vi "Single Class_Multiple_State_External [].vi"(0 "State#":i32=1000, 1 "State_Interval_Time(s)":dbl=0.001 min=0.0 max=86400.0 format="%#_13p", 2 "Time Target (s)":dbl=30.0 format="%#_13g", 3 "System_Delay(s)":dbl=0.01 min=0.0 max=86400.0 format="%#_13p") -> ()   [LabVIEW 2021]
uses:
  C:/Program Files (x86)/Hyper State Machine Framework/SSW_Hyper_State_Machine.lvlibp/State_Machine_Class/Main_State_Machine/Hyper_State_Machine.lvclass
  C:/Program Files (x86)/Hyper State Machine Framework/SSW_Hyper_State_Machine.lvlibp/State_Machine_Class/State_Machine_Module.llb/State Machine[].ctl
  C:/Program Files (x86)/Hyper State Machine Framework/SSW_Hyper_State_Machine.lvlibp/State_Machine_Class/State_Machine_Module.llb/Iterval.ctl
  C:/Program Files (x86)/Hyper State Machine Framework/SSW_Hyper_State_Machine.lvlibp/State_Machine_Class/State_Machine_Module.llb/Lock_Unlock.ctl
  C:/Program Files (x86)/Hyper State Machine Framework/SSW_Hyper_State_Machine.lvlibp
panel:
  in  "State[]":refnum<class "Hyper_State_Machine.lvclass">[](array[class])
  out "Current State":string
  out "Show_Stop_Button":bool=TRUE
  in  "Unlock":bool
  in  "Reset":bool
  in  "Lock Even":bool
  in  "Lock Odd":bool
  in  "lock All":bool
  in  "Stop":bool
  out "Timing":dbl[](array[numeric])
  out "Lock":bool[](array[boolean])
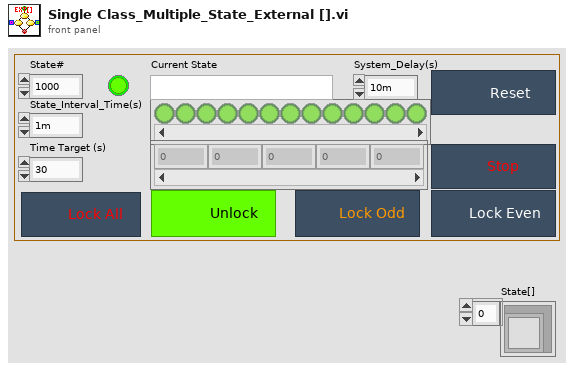
[diagram p1: front panel]
types:
  T1 = typedef "SSW_Hyper_State_Machine.lvlibp/State Machine.ctl" = cluster{"Command":string, "Data":variant}
  T2 = typedef "SSW_Hyper_State_Machine.lvlibp/State Machine[].ctl" = cluster{"Command":string, "Data":variant}[]
  T3 = typedef "SSW_Hyper_State_Machine.lvlibp/Lock_Unlock.ctl" = cluster{"Action_Mode (Get)":enum16{"Set", "Get"}, "Action_Set (False)":bool, "State_In (Wait)":string}
  T4 = typedef "SSW_Hyper_State_Machine.lvlibp/Iterval.ctl" = cluster{"Delay(s)":dbl, "State (Interval_Delay)":string}
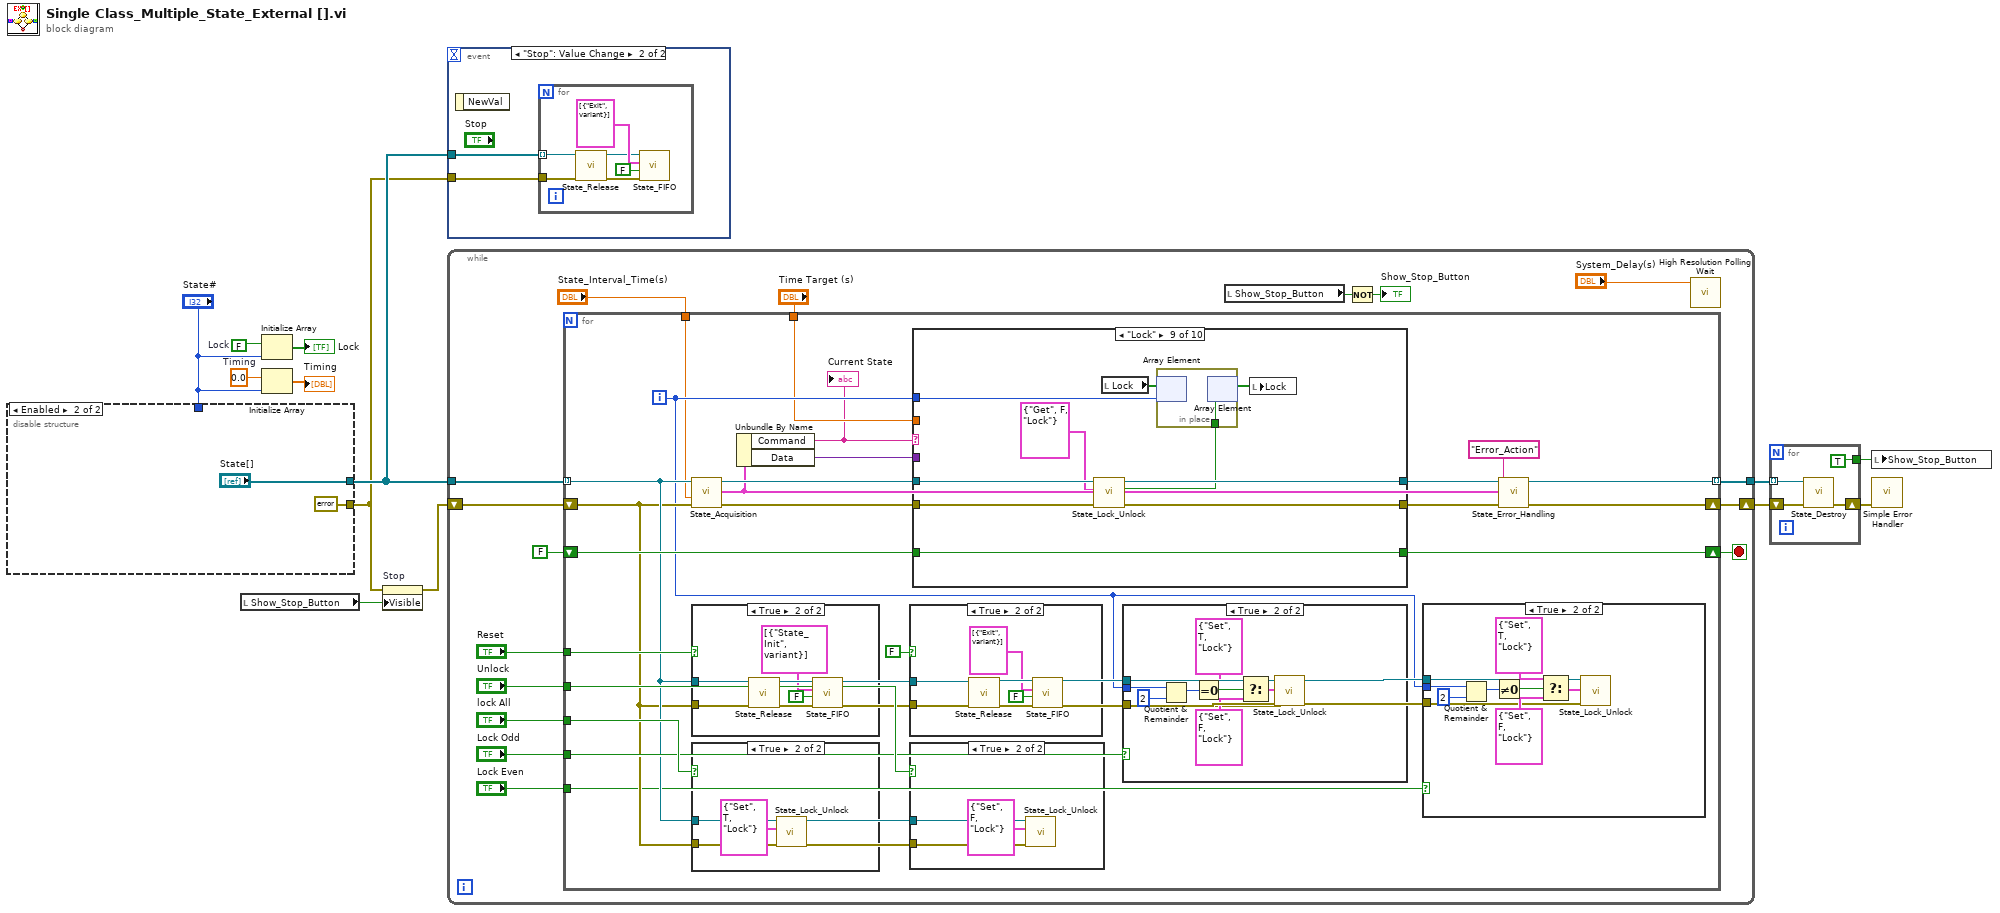
[diagram p0: block diagram]
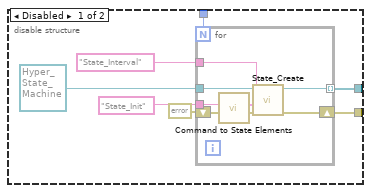
[diagram p2: hidden frame]
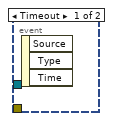
[diagram p3: hidden frame]
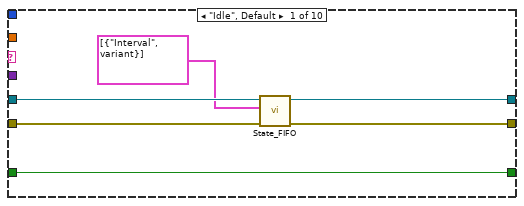
[diagram p10: hidden frame]
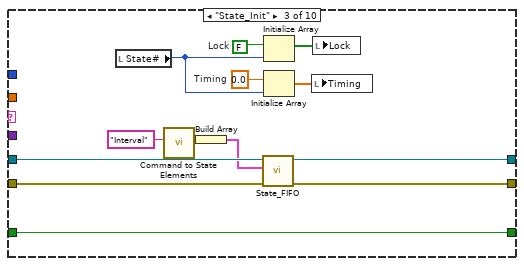
[diagram p12: hidden frame]
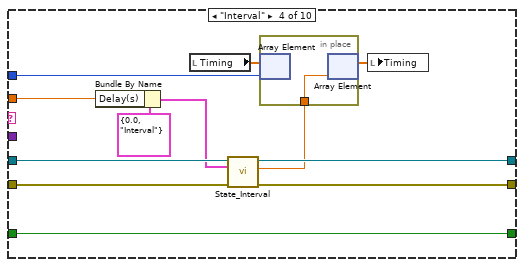
[diagram p13: hidden frame]
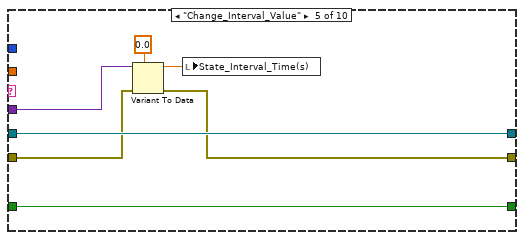
[diagram p14: hidden frame]
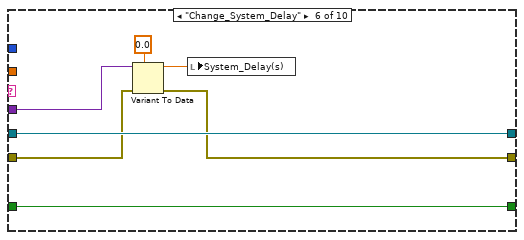
[diagram p15: hidden frame]
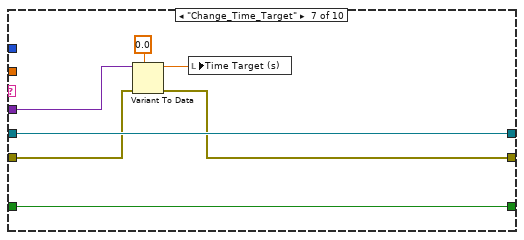
[diagram p16: hidden frame]
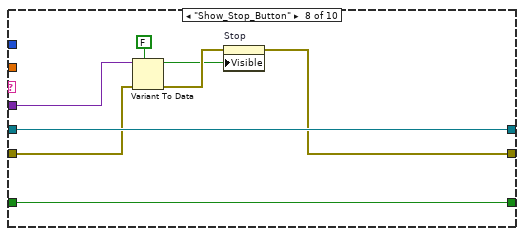
[diagram p17: hidden frame]
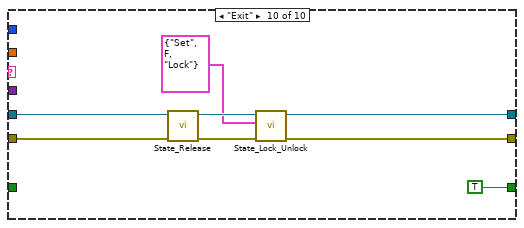
[diagram p18: hidden frame]
diagram:
  w10 = 0.0  # Timing
  w13 = FALSE  # Lock
  n1 = disable-structure shown="Enabled" {
    disable-tunnel: "State#" -> [w20 _]
    disable-tunnel: [w19 "State[]"] -> w2
    disable-tunnel: [w18 errorcluster {"status"=FALSE, "code"=0, "source"=""} ("error out")] -> w1
    frame Disabled {
      n2 = for {
        N: w20 -> [_]
        tunnel: refnum<class "Hyper_State_Machine.lvclass"> refnum ("SSW_Hyper_State_Machine.lvlibp:Hyper_State_Machine.lvclass") -> [w27]
        tunnel: "State_Init" ("Command") -> [w25]
        tunnel: "State_Interval" ("Core_Interval_Name(State_Interval)") -> [w24]
        shift-right: [w23] -> w18
        shift-left: errorcluster {"status"=FALSE, "code"=0, "source"=""} ("error out") -> [w22]
        tunnel: [w21] -> w19 mode=indexing
        n3 = call "Command to State Elements.vi"("Command"=w25) -> ("Command to State Elements"=w26:T1)  [unwired: 10 in]
        n4 = call-dynamic "State_Create.vi"("error in (no error)"=w22, "Init_State(Option)"=w26, "State_Interval_Name"=w24, "State_Machine_Class in"=w27) -> ("error out"=w23:errorcluster, "State_Machine_Class out"=w21:refnum<class "Hyper_State_Machine.lvclass">)  [unwired: 5 in, 1 out]
      }
    }
    frame Enabled {
    }
  }
  n5 = local read "Show_Stop_Button"() -> (w4:bool)
  n6 = Initialize Array(w13, "State#") -> (→"Lock":bool[])
  n7 = Initialize Array(w10, "State#") -> (→"Timing":dbl[])
  n8 = property on="Stop" class="Bool"(error in=w1, "Visible"=w4) -> (error out=w5:errorcluster)  [unwired: 1 in, 1 out]
  n9 = event shown="[1] \"Stop\": Value Change" {
    selector: _ -> [_ _]
    dyn-events: _ -> [_ _]
    timeout: _ -> [_ _]
    tunnel: w2 -> [_ w31]
    tunnel: w1 -> [_ w30]
    event Timeout {
      n10 = event-data() -> ()  [unwired: 1 in, 3 out]
    }
    event "Stop": Value Change {
      n11 = event-data() -> ()  [unwired: 1 in, 1 out]
      n12 = for {
        tunnel: w31 -> [w33] mode=indexing
        tunnel: w30 -> [w32]
        n13 = call-dynamic "State_Release.vi"("error in (no error)"=w32, "State_Machine_Class in"=w33) -> ("error out"=w35:errorcluster, "State_Machine_Class out"=w34:refnum<class "Hyper_State_Machine.lvclass">)  [unwired: 8 in]
        n14 = call-dynamic "State_FIFO.vi"("error in (no error)"=w35, "State_Interval(Enable)"=FALSE, "State Machine[]"=T2 [{"Command"="Exit", "Data"=variant}], "State_Machine_Class in"=w34) -> ()  [unwired: 6 in, 2 out]
      }
    }
  }
  n15 = while {
    tunnel: w2 -> [w53]
    tunnel: [w49] -> w7
    shift-right: [w48] -> w6
    shift-left: w5 -> [w52]
    stop <- w51 stop-if-true
    n16 = for {
      tunnel: w53 -> [w61] mode=indexing
      shift-right: [w73] -> w48
      shift-left: w52 -> [w60]
      shift-right: [w68] -> w51
      shift-left: FALSE -> [w67]
      tunnel: [w66] -> w49 mode=indexing
      tunnel: "Reset" -> [w65]
      tunnel: "lock All" -> [w64]
      tunnel: "Unlock" -> [w63]
      tunnel: "Lock Odd" -> [w62]
      tunnel: "Lock Even" -> [w59]
      tunnel: "Time Target (s)" -> [w57]
      tunnel: "State_Interval_Time(s)" -> [w56]
      i -> [w58]
      n17 = call-dynamic "State_Acquisition.vi"("error in (no error)"=w60, "State_Interval_Time(s)"=w56, "Main_Machine_State_Class in"=w61) -> ("error out"=w74:errorcluster, "State"=w72:T1, "Main_Machine_State_Class out"=w75:refnum<class "Hyper_State_Machine.lvclass">)  [unwired: 2 in, 4 out]
      n18 = case shown="True" w65 {
        tunnel: w61 -> [_ w112]
        tunnel: w60 -> [_ w108]
        frame False {
        }
        frame True {
          n19 = call-dynamic "State_Release.vi"("error in (no error)"=w108, "State_Machine_Class in"=w112) -> ("error out"=w110:errorcluster, "State_Machine_Class out"=w111:refnum<class "Hyper_State_Machine.lvclass">)  [unwired: 8 in]
          n20 = call-dynamic "State_FIFO.vi"("error in (no error)"=w110, "State_Interval(Enable)"=FALSE, "State Machine[]"=T2 [{"Command"="State_Init", "Data"=variant}], "State_Machine_Class in"=w111) -> ()  [unwired: 6 in, 2 out]
        }
      }
      n21 = case shown="True" w64 {
        tunnel: w61 -> [_ w100]
        tunnel: w60 -> [_ w99]
        frame False {
        }
        frame True {
          n22 = call-dynamic "State_Lock_Unlock.vi"("error in (no error)"=w99, "Parameter"=T3 {"Action_Mode (Get)"=enum."Set", "Action_Set (False)"=TRUE, "State_In (Wait)"="Lock"}, "State_Machine_Class in"=w100) -> ()  [unwired: 6 in, 3 out]
        }
      }
      n23 = Unbundle By Name(w72) -> ("Command"=w54:string, "Data"=w76:variant)
      "Current State" <- w54
      n24 = case shown="True" FALSE {
        tunnel: w61 -> [_ w106]
        tunnel: w60 -> [_ w102]
        frame False {
        }
        frame True {
          n25 = call-dynamic "State_Release.vi"("error in (no error)"=w102, "State_Machine_Class in"=w106) -> ("error out"=w104:errorcluster, "State_Machine_Class out"=w105:refnum<class "Hyper_State_Machine.lvclass">)  [unwired: 8 in]
          n26 = call-dynamic "State_FIFO.vi"("error in (no error)"=w104, "State_Interval(Enable)"=FALSE, "State Machine[]"=T2 [{"Command"="Exit", "Data"=variant}], "State_Machine_Class in"=w105) -> ()  [unwired: 6 in, 2 out]
        }
      }
      n27 = case shown="True" w63 {
        tunnel: w61 -> [_ w96]
        tunnel: w60 -> [_ w97]
        frame False {
        }
        frame True {
          n28 = call-dynamic "State_Lock_Unlock.vi"("error in (no error)"=w97, "Parameter"=T3 {"Action_Mode (Get)"=enum."Set", "Action_Set (False)"=FALSE, "State_In (Wait)"="Lock"}, "State_Machine_Class in"=w96) -> ()  [unwired: 6 in, 3 out]
        }
      }
      n29 = case shown="\"Lock\"" w54 {
        tunnel: w76 -> [_ _ _ _ w153 w160 w167 w175 _ _]
        tunnel: w75 -> [w117 w121 w133 w140 w154 w161 w168 w176 w186 w194]
        tunnel: w74 -> [w116 w120 w131 w139 w152 w159 w166 w174 w185 w193]
        tunnel: [w115 w121 w132 w137 w154 w161 w168 w176 w184 w190] -> w70
        tunnel: [w114 w120 w130 w136 w151 w158 w165 w169 w183 w189] -> w69
        tunnel: w58 -> [_ _ _ w146 _ _ _ _ w178 _]
        tunnel: [w118 w119 w134 w143 w149 w156 w163 w173 w181 TRUE] -> w68
        tunnel: w67 -> [w118 w119 w134 w143 w149 w156 w163 w173 w181 _]
        tunnel: w57 -> [_ _ _ w142 _ _ _ _ _ _]
        frame "Idle", Default {
          n30 = call-dynamic "State_FIFO.vi"("error in (no error)"=w116, "State Machine[]"=T2 [{"Command"="Interval", "Data"=variant}], "State_Machine_Class in"=w117) -> ("error out"=w114:errorcluster, "State_Machine_Class out"=w115:refnum<class "Hyper_State_Machine.lvclass">)  [unwired: 7 in]
        }
        frame "State_Interval" {
          # "Execute Every Define of State Interval Time"
        }
        frame "State_Init" {
          w126 = 0.0  # Timing
          w125 = FALSE  # Lock
          n31 = local read "State#"() -> (w124:i32)
          n32 = call "Command to State Elements.vi"("Command"="Interval") -> ("Command to State Elements"=w128:T1)  [unwired: 10 in]
          n33 = Build Array(w128) -> (w127:T1[])
          n34 = call-dynamic "State_FIFO.vi"("error in (no error)"=w131, "State Machine[]"=w127, "State_Machine_Class in"=w133) -> ("error out"=w130:errorcluster, "State_Machine_Class out"=w132:refnum<class "Hyper_State_Machine.lvclass">)  [unwired: 7 in]
          n35 = Initialize Array(w125, w124) -> (w122:bool[])
          n36 = Initialize Array(w126, w124) -> (w123:dbl[])
          n37 = local write "Timing"(w123) -> ()
          n38 = local write "Lock"(w122) -> ()
        }
        frame "Interval" {
          n39 = Bundle By Name(cluster=T4 {"Delay(s)"=0.0, "State (Interval_Delay)"="Interval"} ("Parameter"), "Delay(s)"=w142) -> (w138:T4)
          n40 = local read "Timing"() -> (w145:dbl[])
          n41 = call-dynamic "State_Interval.vi"("error in (no error)"=w139, "Parameter"=w138, "State_Machine_Class in"=w140) -> ("error out"=w136:errorcluster, "Elapsed Time(s)"=w135:dbl, "State_Machine_Class out"=w137:refnum<class "Hyper_State_Machine.lvclass">)  [unwired: 6 in]
          n42 = in-place {
            in-place-border: w135 -> [w147]
            n43 = in-place-array #1(w145, w146) -> ()  [unwired: 1 out]
            n44 = in-place-array #1(w147) -> (w144:dbl[])  [unwired: 1 out]
          }
          n45 = local write "Timing"(w144) -> ()
        }
        frame "Change_Interval_Value" {
          n46 = Variant To Data(error in=w152, type=0.0 ("Time Target (s)"), Variant=w153) -> (data=w148:dbl, error out=w151:errorcluster)
          n47 = local write "State_Interval_Time(s)"(w148) -> ()
        }
        frame "Change_System_Delay" {
          n48 = Variant To Data(error in=w159, type=0.0 ("Time Target (s)"), Variant=w160) -> (data=w155:dbl, error out=w158:errorcluster)
          n49 = local write "System_Delay(s)"(w155) -> ()
        }
        frame "Change_Time_Target" {
          n50 = Variant To Data(error in=w166, type=0.0 ("Time Target (s)"), Variant=w167) -> (data=w162:dbl, error out=w165:errorcluster)
          n51 = local write "Time Target (s)"(w162) -> ()
        }
        frame "Show_Stop_Button" {
          n52 = Variant To Data(error in=w174, type=FALSE, Variant=w175) -> (data=w170:bool, error out=w171:errorcluster)
          n53 = property on="Stop" class="Bool"(error in=w171, "Visible"=w170) -> (error out=w169:errorcluster)  [unwired: 1 in, 1 out]
        }
        frame "Lock" {
          n54 = call-dynamic "State_Lock_Unlock.vi"("error in (no error)"=w185, "Parameter"=T3 {"Action_Mode (Get)"=enum."Get", "Action_Set (False)"=FALSE, "State_In (Wait)"="Lock"}, "State_Machine_Class in"=w186) -> ("error out"=w183:errorcluster, "Action_Get"=w177:bool, "State_Machine_Class out"=w184:refnum<class "Hyper_State_Machine.lvclass">)  [unwired: 6 in]
          n55 = local read "Lock"() -> (w179:bool[])
          n56 = in-place {
            in-place-border: w177 -> [w187]
            n57 = in-place-array #2(w179, w178) -> ()  [unwired: 1 out]
            n58 = in-place-array #2(w187) -> (w180:bool[])  [unwired: 1 out]
          }
          n59 = local write "Lock"(w180) -> ()
        }
        frame "Exit" {
          n60 = call-dynamic "State_Release.vi"("error in (no error)"=w193, "State_Machine_Class in"=w194) -> ("error out"=w191:errorcluster, "State_Machine_Class out"=w192:refnum<class "Hyper_State_Machine.lvclass">)  [unwired: 8 in]
          n61 = call-dynamic "State_Lock_Unlock.vi"("error in (no error)"=w191, "Parameter"=T3 {"Action_Mode (Get)"=enum."Set", "Action_Set (False)"=FALSE, "State_In (Wait)"="Lock"}, "State_Machine_Class in"=w192) -> ("error out"=w189:errorcluster, "State_Machine_Class out"=w190:refnum<class "Hyper_State_Machine.lvclass">)  [unwired: 6 in, 1 out]
        }
      }
      n62 = case shown="True" w62 {
        tunnel: w58 -> [_ w88]
        tunnel: w61 -> [_ w87]
        tunnel: w60 -> [_ w86]
        frame False {
        }
        frame True {
          n63 = Quotient & Remainder(x=w88, y=2) -> (x-y*floor(x/y)=w93:i32)  [unwired: 1 out]
          n64 = Equal To 0?(x=w93) -> (x = 0?=w92:bool)
          n65 = Select(t=T3 {"Action_Mode (Get)"=enum."Set", "Action_Set (False)"=TRUE, "State_In (Wait)"="Lock"} ("Parameter"), s=w92, f=T3 {"Action_Mode (Get)"=enum."Set", "Action_Set (False)"=FALSE, "State_In (Wait)"="Lock"} ("Parameter")) -> (s? t:f=w89:T3)
          n66 = call-dynamic "State_Lock_Unlock.vi"("error in (no error)"=w86, "Parameter"=w89, "State_Machine_Class in"=w87) -> ()  [unwired: 6 in, 3 out]
        }
      }
      n67 = case shown="True" w59 {
        tunnel: w58 -> [_ w79]
        tunnel: w61 -> [_ w78]
        tunnel: w60 -> [_ w77]
        frame False {
        }
        frame True {
          n68 = Quotient & Remainder(x=w79, y=2) -> (x-y*floor(x/y)=w84:i32)  [unwired: 1 out]
          n69 = Not Equal To 0?(x=w84) -> (x != 0?=w83:bool)
          n70 = Select(t=T3 {"Action_Mode (Get)"=enum."Set", "Action_Set (False)"=TRUE, "State_In (Wait)"="Lock"} ("Parameter"), s=w83, f=T3 {"Action_Mode (Get)"=enum."Set", "Action_Set (False)"=FALSE, "State_In (Wait)"="Lock"} ("Parameter")) -> (s? t:f=w80:T3)
          n71 = call-dynamic "State_Lock_Unlock.vi"("error in (no error)"=w77, "Parameter"=w80, "State_Machine_Class in"=w78) -> ()  [unwired: 6 in, 3 out]
        }
      }
      n72 = call-dynamic "State_Error_Handling.vi"("error in (no error)"=w69, "Reply_State_Name"="Error_Action", "Handling_State(State_Acquisition)"=w72, "State_Machine_Class in"=w70) -> ("error out"=w73:errorcluster, "State_Machine_Class out"=w66:refnum<class "Hyper_State_Machine.lvclass">)  [unwired: 6 in]
    }
    n73 = local read "Show_Stop_Button"() -> (w39:bool)
    n74 = Not(x=w39) -> (.not. x?=→"Show_Stop_Button":bool)
    n75 = call <vilib>:"High Resolution Polling Wait.vi"("seconds to wait"="System_Delay(s)") -> ()  [unwired: 10 in, 1 out]
  }
  n76 = for {
    shift-right: [w199] -> w8
    shift-left: w6 -> [w198]
    tunnel: w7 -> [w197] mode=indexing
    tunnel: [TRUE ("Show_Stop_Button")] -> w3
    n77 = call-dynamic "State_Destroy.vi"("error in (no error)"=w198, "State_Machine_Class in"=w197) -> ("error out"=w199:errorcluster)  [unwired: 9 in]
  }
  n78 = local write "Show_Stop_Button"(w3) -> ()
  n79 = call <vilib>:"Simple Error Handler.vi"("error in (no error)"=w8) -> ()  [unwired: 4 in, 5 out]
